vi "update-screen-values.vi"(8 "error in (no error)":errorcluster, 9 "Array":string[](array[string]), 10 "tags":string[](array[string]), 11 "dbc in":refnum<class "dbc.lvclass">) -> (0 "error out":errorcluster, 3 "dbc out":refnum<class "dbc.lvclass">)   [LabVIEW 2015, in "dbc.lvclass"]
uses:
  dbc.lvclass
  dbc.lvclass/dbc.ctl
  read-tree-ref.vi
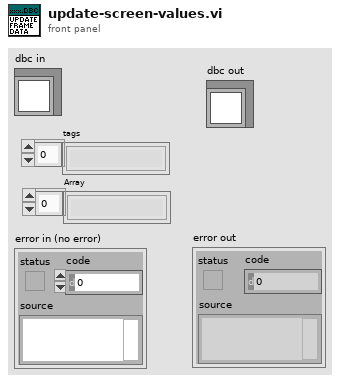
[diagram p1: front panel]
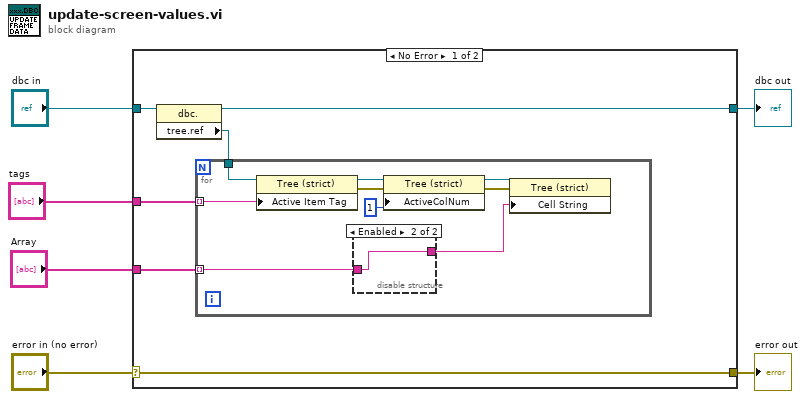
[diagram p0: block diagram]
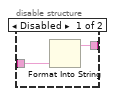
[diagram p2: hidden frame]
diagram:
  n1 = case shown="No Error" "error in (no error)" {
    selector: "error in (no error)" -> [w11 w26]
    tunnel: [w11 w26] -> w5
    tunnel: [w10 w25] -> w3
    tunnel: "dbc in" -> [w12 w25]
    tunnel: "tags" -> [w8 _]
    tunnel: "Array" -> [w7 _]
    frame No Error {
      n2 = property class="dbc."(reference=w12) -> (reference out=w10:refnum<class "dbc.lvclass">, "tree.ref"=w9:refnum<vi>)  [unwired: 1 in, 1 out]
      n3 = for {
        tunnel: w9 -> [w16]
        tunnel: w8 -> [w15] mode=indexing
        tunnel: w7 -> [w14] mode=indexing
        n4 = property class="Tree (strict)"(reference=w16, "Active Item Tag"=w15) -> (reference out=w19:refnum<vi>, error out=w18:errorcluster)  [unwired: 1 in]
        n5 = disable-structure shown="Enabled" {
          disable-tunnel: w14 -> [w23 w24]
          disable-tunnel: [w22 w24] -> w13
          frame Disabled {
            n6 = Format Into String(w23) -> (resulting string=w22:string)  [unwired: 3 in, 1 out]
          }
          frame Enabled {
          }
        }
        n7 = property class="Tree (strict)"(reference=w19, error in=w18, "ActiveColNum"=1 ("Active Cell:Active Column Number")) -> (reference out=w21:refnum<vi>, error out=w17:errorcluster)
        n8 = property class="Tree (strict)"(reference=w21, error in=w17, "Cell String"=w13) -> ()  [unwired: 2 out]
      }
    }
    frame Error {
    }
  }
  "error out" <- w5
  "dbc out" <- w3
